vi "电源管理UI.vi"() -> ()   [LabVIEW 2016, in "环境动力单元.lvlib"]
uses:
  <vilib>/Utility/miscctls.llb/LVPointTypeDef.ctl
  <vilib>/Plasmionique/MB Master/MB_Master/MB_Master.lvclass
  <vilib>/Utility/config.llb/NI_LVConfig.lvlib
  <vilib>/ptbypt/NI_PtbyPt.lvlib
  API/AIRMAR WeatherCaster/AIRMAR WeatherCaster.lvlib
panel:
  out "门禁2状态":bool
  in  "停止":bool
  out "运行状态":string
  in  "采配水单次启动":bool
  out "充放电信息 2":T1 caption="充放电信息_KWH" {"总累计充电量" format="%.2f"; "当年累计充电量" format="%.2f"; "当月累计充电量" format="%.2f"; "当日累计充电量" format="%.2f"; "当年累计用电量" format="%.2f"; "当月累计用电量" format="%.2f"; "当日累计用电量" format="%.2f"}
  out "状态 2":string caption="状态"
  out "状态":string
  out "充放电信息":T1 caption="充放电信息_KWH" {"总累计充电量" format="%.2f"; "当年累计充电量" format="%.2f"; "当月累计充电量" format="%.2f"; "当日累计充电量" format="%.2f"; "当年累计用电量" format="%.2f"; "当月累计用电量" format="%.2f"; "当日累计用电量" format="%.2f"}
  out "通讯状态 3":bool
  out "通讯状态 2":bool
  out "通讯状态":bool
  in  "排气扇设置":bool
  in  "冰箱设置":bool
  in  "采配水设置":bool caption="报警设置"
  in  "MPPT-24 串口":refnum<visa-resource-name> caption="MPPT-24"
  in  "MPPT-24 启用":bool
  in  "MPPT-12 串口":refnum<visa-resource-name> caption="MPPT-12"
  in  "MPPT-12 启用":bool
  in  "报警设置":bool
  in  "排气扇":bool
  in  "冰箱":bool
  in  "排液阀":bool
  in  "采水泵":bool
  out "控制器信息 2":cluster{"设备温度℃":dbl} caption="控制器信息"
  out "直流负载信息 2":cluster{"负载电压V":dbl, "负载电流A":dbl, "负载功率W":dbl} caption="直流负载信息"
  out "蓄电池信息 2":T2 caption="蓄电池信息"
  out "阵列信息 2":cluster{"阵列电压V":dbl, "阵列电流A":dbl, "发电功率W":dbl} caption="阵列信息"
  out "控制器信息":cluster{"设备温度℃":dbl}
  out "直流负载信息":cluster{"负载电压V":dbl, "负载电流A":dbl, "负载功率W":dbl}
  out "蓄电池信息":T2
  out "阵列信息":cluster{"阵列电压V":dbl, "阵列电流A":dbl, "发电功率W":dbl}
  out "湿度":dbl format="%.0f %%RH"
  out "室温":dbl format="%.2f ℃"
  out "液位状态":bool
  out "门禁1状态":bool
  out "烟雾报警":bool
  out "水浸报警":bool
  in  "ZLAN启用":bool
  in  "模拟量配置":bool
  # "监控信息"
  # "MPPT-12"
  # "MPPT-24"
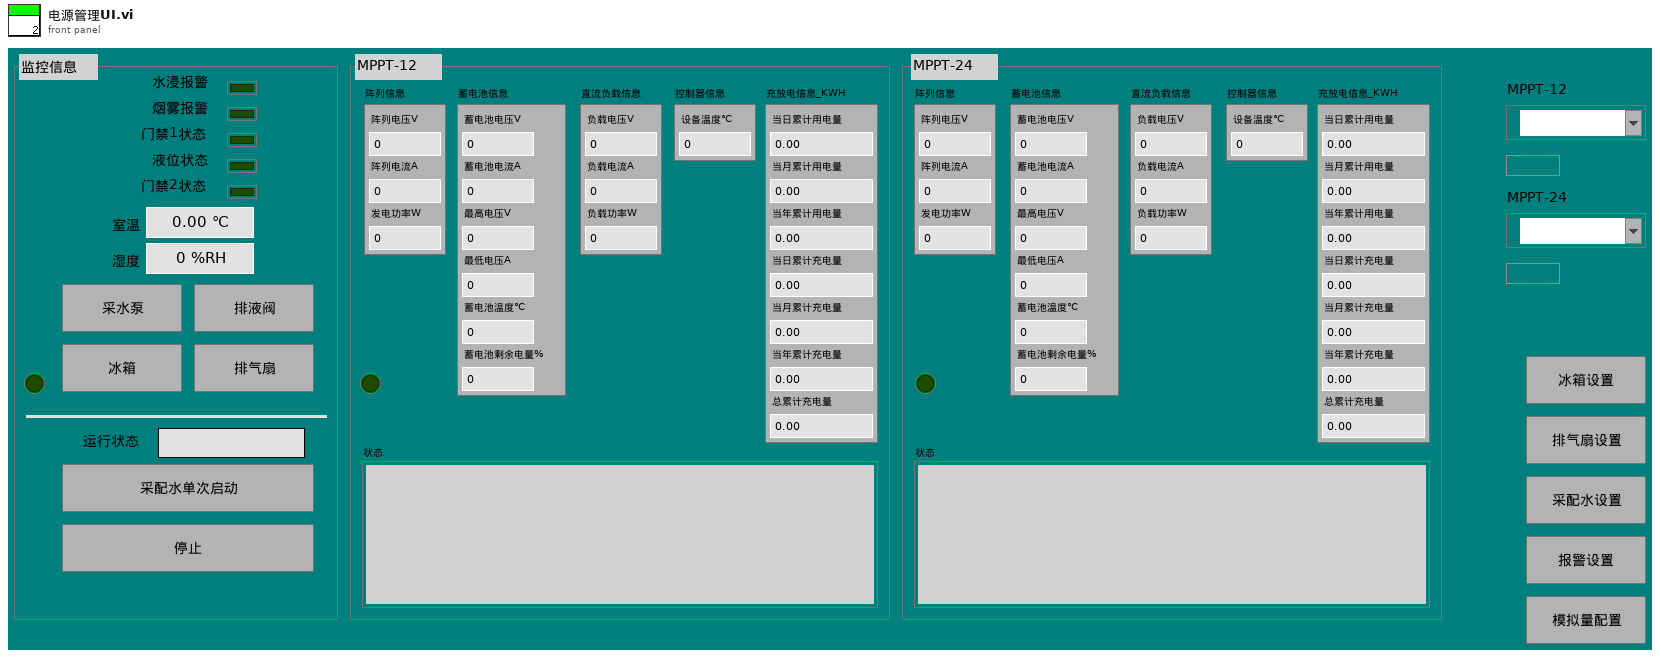
[diagram p1: front panel]
types:
  T1 = cluster{"当日累计用电量":sgl, "当月累计用电量":sgl, "当年累计用电量":sgl, "当日累计充电量":sgl, "当月累计充电量":sgl, "当年累计充电量":sgl, "总累计充电量":sgl}
  T2 = cluster{"蓄电池电压V":dbl, "蓄电池电流A":dbl, "最高电压V":dbl, "最低电压A":dbl, "蓄电池温度℃":dbl, "蓄电池剩余电量%":dbl}
  T3 = typedef "LVPointTypeDef.ctl" = cluster{"Horizontal":i16, "Vertical":i16}
  T4 = cluster{"蓄电池电压":dbl, "室温":dbl, "湿度":dbl, "水浸报警":bool, "烟雾报警":bool, "门禁1状态":bool, "门禁2状态":bool}
  T5 = cluster{"AD0":dbl, "AD1":dbl, "AD2":dbl, "AD3":dbl, "AD4":dbl, "AD5":dbl, "AD6":dbl, "AD7":dbl}
  T6 = typedef "NI_LVConfig.lvlib/Config Data RefNum.ctl" = refnum<k1>
  T7 = cluster{"时间":timestamp, "阵列电压_V":dbl, "阵列电流_A":dbl, "发电功率_W":dbl, "蓄电池电压_V":dbl, "蓄电池电流_A":dbl, "最高电压_V":dbl, "最低电压_A":dbl, "蓄电池温度_℃":dbl, "蓄电池剩余电量_%":dbl, "负载电压_V":dbl, "负载电流_A":dbl, "负载功率_W":dbl, "设备温度_℃":dbl, "当日累计用电量_KWH":dbl, "当月累计用电量_KWH":dbl, "当年累计用电量_KWH":dbl, "当日累计充电量_KWH":dbl, "当月累计充电量_KWH":dbl, "当年累计充电量_KWH":dbl, "总累计充电量_KWH":dbl}
  T8 = typedef "LVDateTimeRec.ctl" = cluster{"秒数的小数部分":dbl, "秒":i32, "分":i32, "时":i32, "日":i32, "月":i32, "年":i32, "天数（周）":i32, "天数（年）":i32, "DST":i32}
  T9 = cluster{"功能开关":enum16{"关闭", "开启"}, "开启时间":u16, "关闭时间":u16}
  T10 = cluster{"功能开关":enum16{"关闭", "开启"}, "排气扇开启温度":dbl, "排气扇关闭温度":dbl}
  T11 = cluster{"原始值最小值":dbl, "原始值最大值":dbl, "转换值最小值":dbl, "转换值最大值":dbl, "原始值最小值 2":dbl, "原始值最大值 2":dbl, "转换值最小值 2":dbl, "转换值最大值 2":dbl, "原始值最小值 3":dbl, "原始值最大值 3":dbl, "转换值最小值 3":dbl, "转换值最大值 3":dbl, "原始值最小值 4":dbl, "原始值最大值 4":dbl, "转换值最小值 4":dbl, "转换值最大值 4":dbl, "原始值最小值 5":dbl, "原始值最大值 5":dbl, "转换值最小值 5":dbl, "转换值最大值 5":dbl, "原始值最小值 6":dbl, "原始值最大值 6":dbl, "转换值最小值 6":dbl, "转换值最大值 6":dbl, "原始值最小值 7":dbl, "原始值最大值 7":dbl, "转换值最小值 7":dbl, "转换值最大值 7":dbl, "原始值最小值 8":dbl, "原始值最大值 8":dbl, "转换值最小值 8":dbl, "转换值最大值 8":dbl}
  T12 = enum8{"Enabled", "Disabled", "Disabled and Grayed Out"}
  T13 = cluster{"Registers[0]":u16, "Registers[1]":u16, "Registers[2]":u16, "Registers[3]":u16, "Registers[4]":u16, "Registers[5]":u16, "Registers[6]":u16, "Registers[7]":u16}
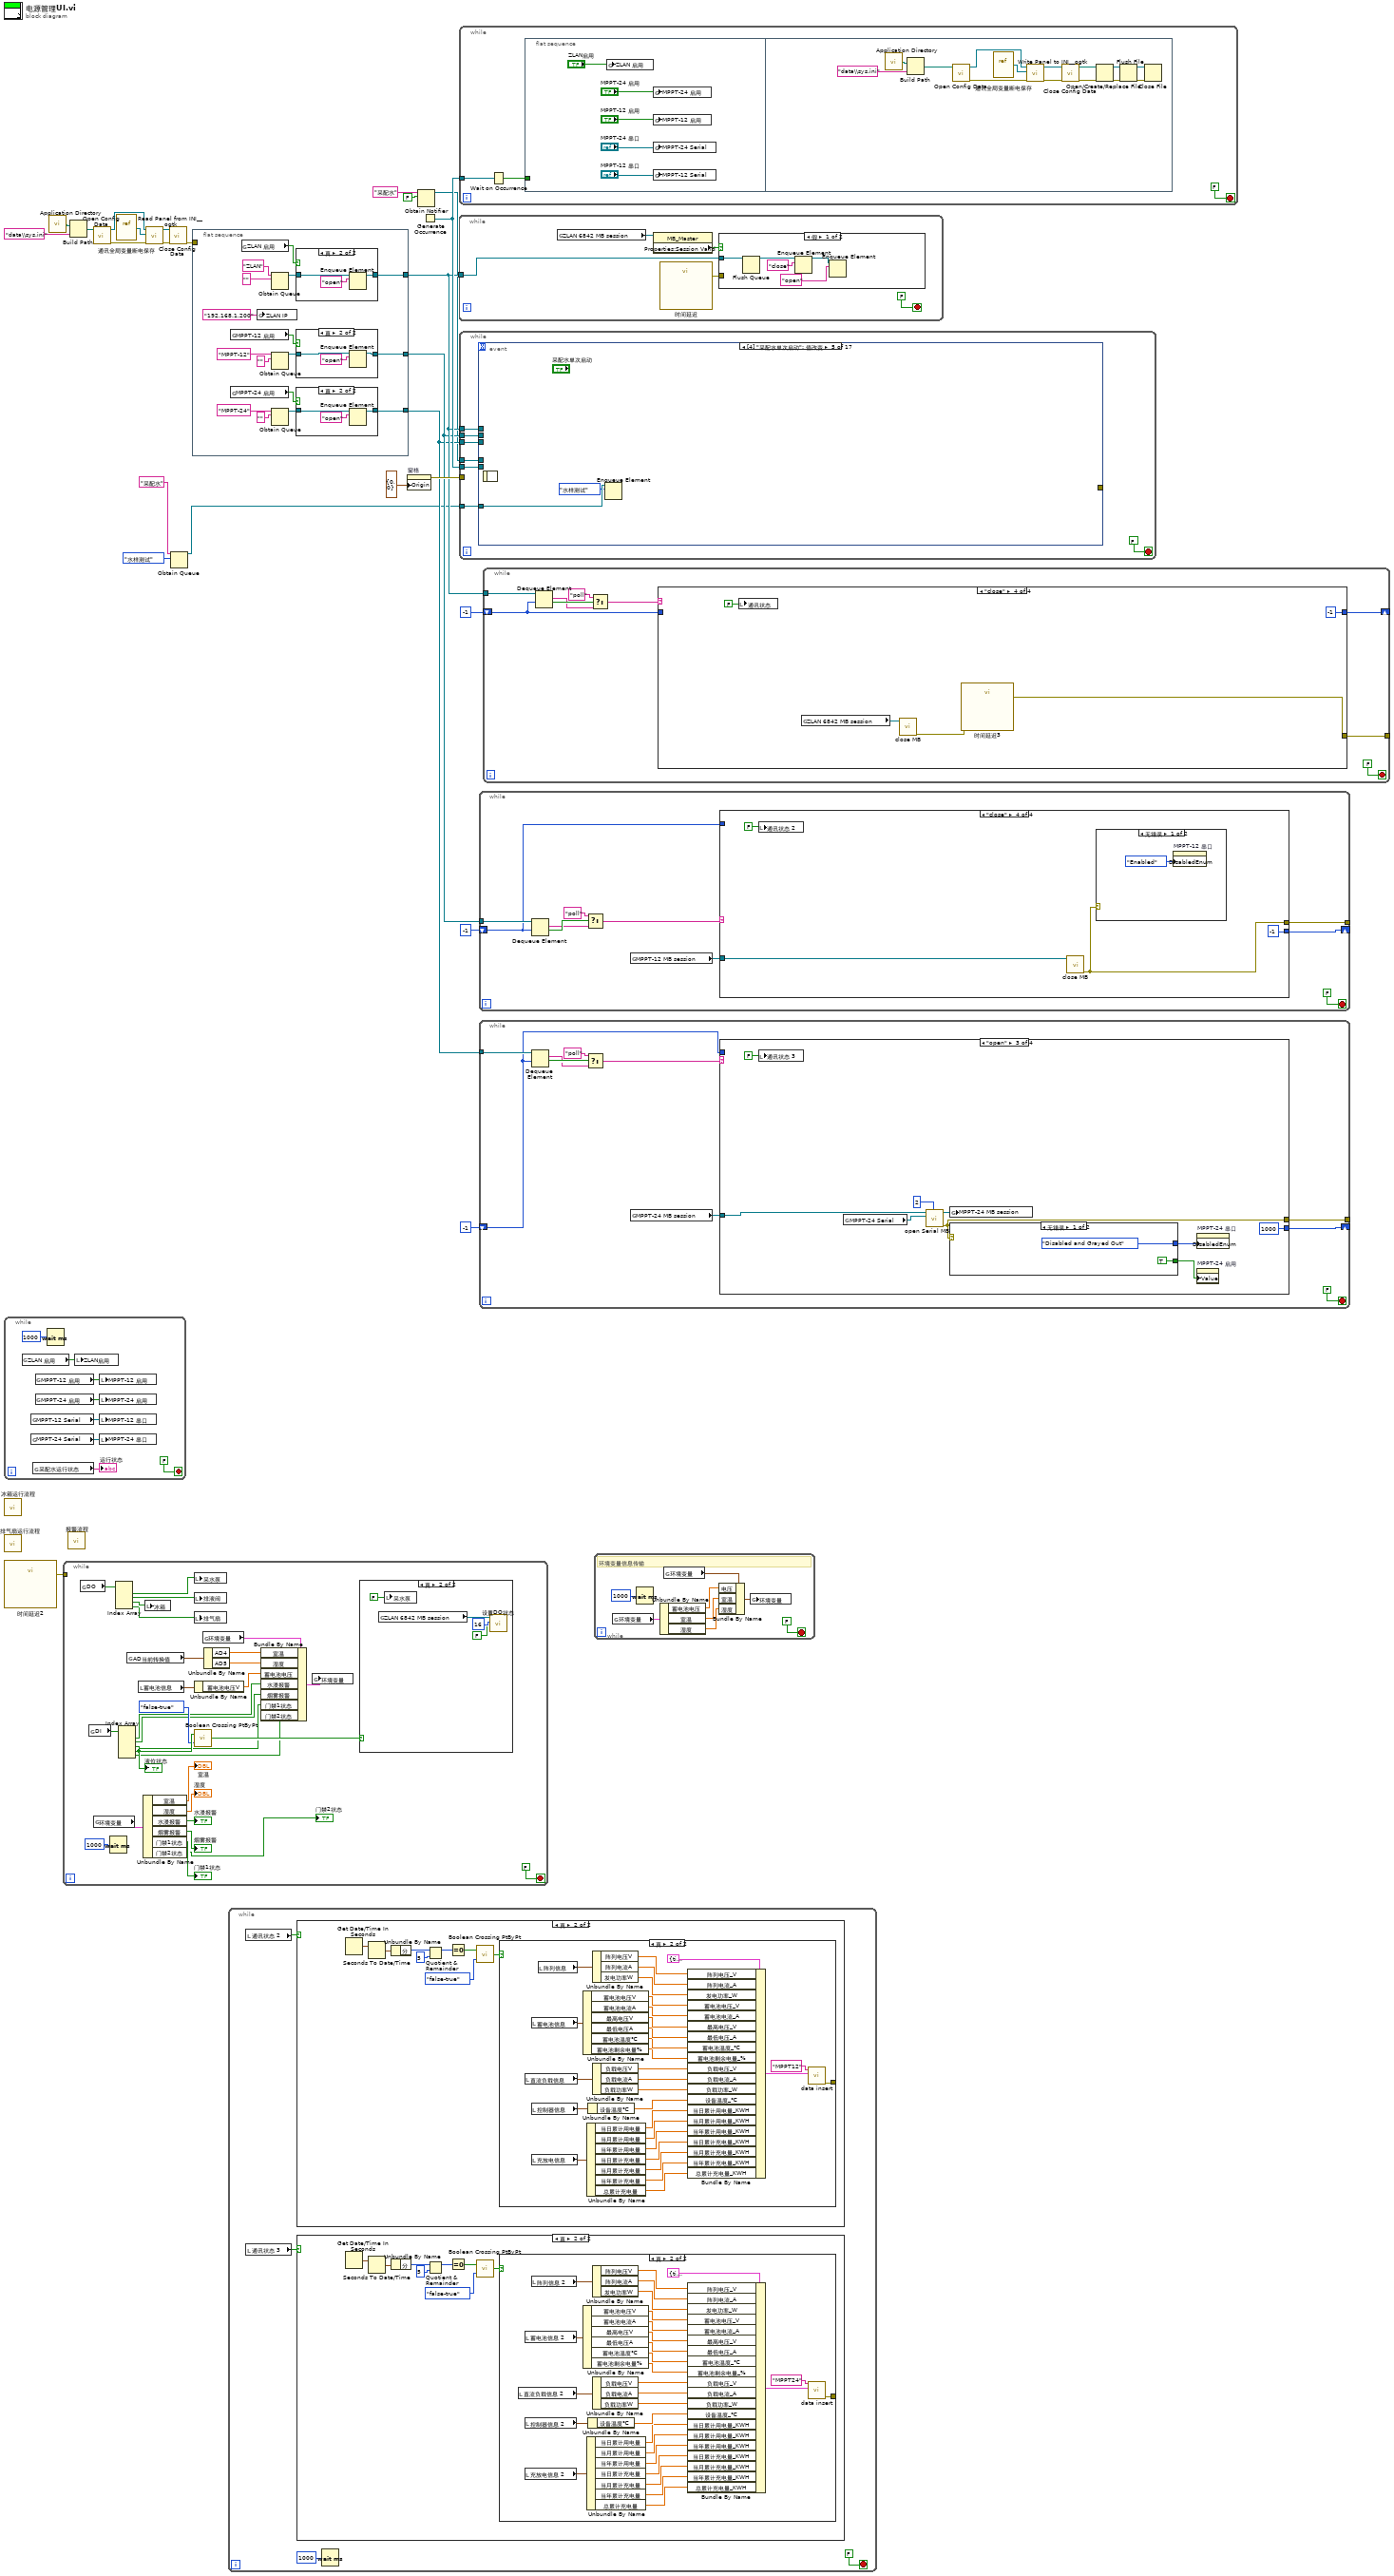
[diagram p0: block diagram]
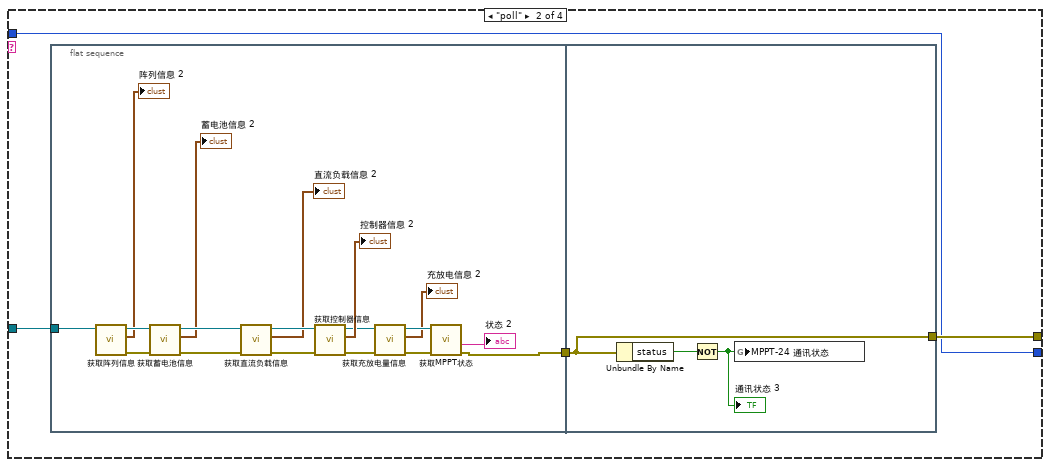
[diagram p7: hidden frame]
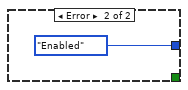
[diagram p8: hidden frame]
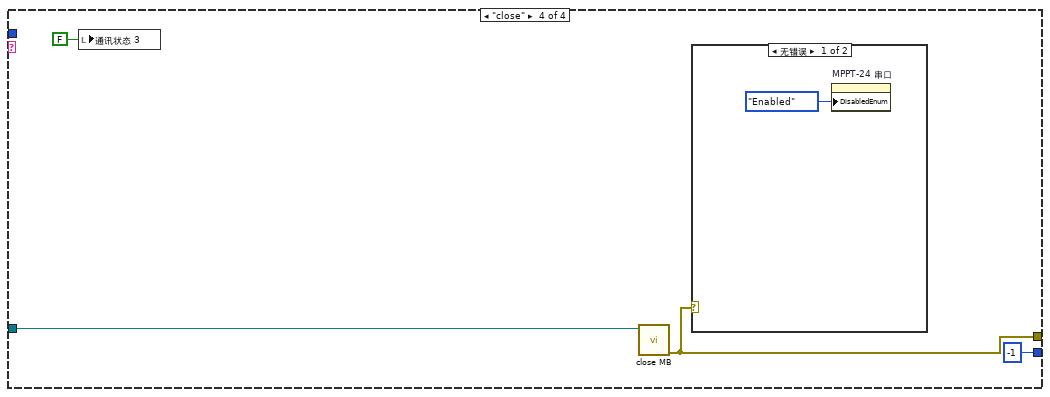
[diagram p9: hidden frame]
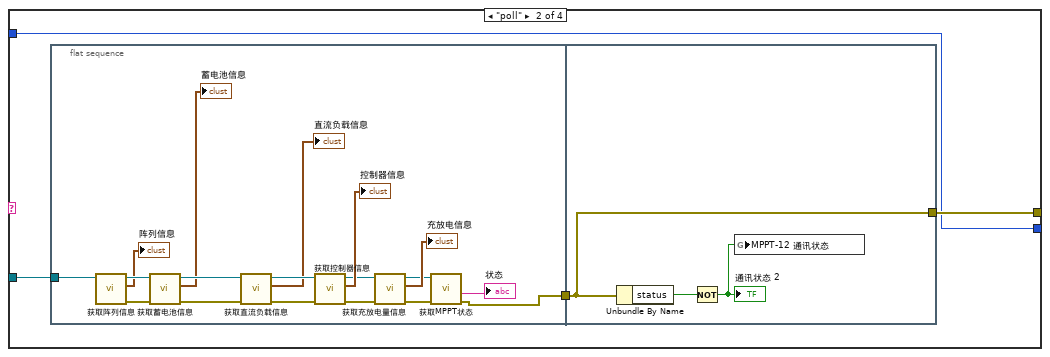
[diagram p12: hidden frame]
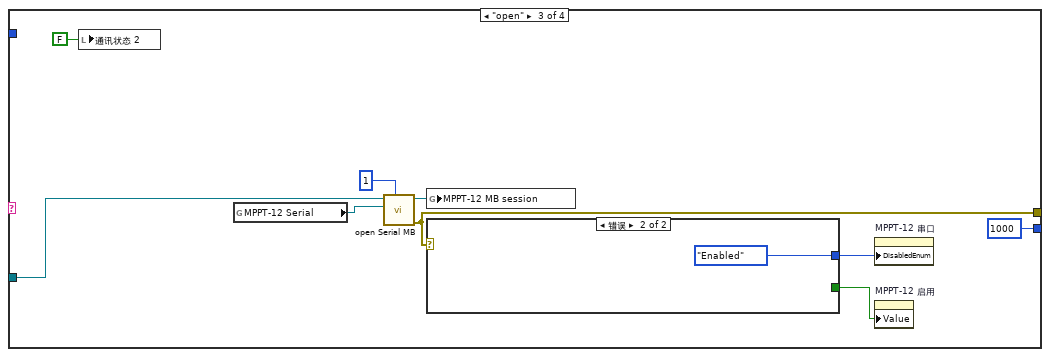
[diagram p13: hidden frame]
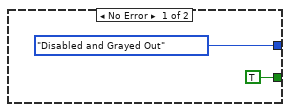
[diagram p14: hidden frame]
diagram:
  n1 = while {
    stop <- FALSE stop-if-true
    n2 = global read "通讯全局变量断电保存.vi" "ZLAN 启用"() -> (w31:bool)
    n3 = global read "通讯全局变量断电保存.vi" "MPPT-12 Serial"() -> (w28:refnum<visa-resource-name>)
    n4 = global read "通讯全局变量断电保存.vi" "MPPT-24 Serial"() -> (w27:refnum<visa-resource-name>)
    n5 = global read "通讯全局变量.vi" "采配水运行状态"() -> (→"运行状态":string)
    n6 = global read "通讯全局变量断电保存.vi" "MPPT-12 启用"() -> (w30:bool)
    n7 = global read "通讯全局变量断电保存.vi" "MPPT-24 启用"() -> (w29:bool)
    n8 = Wait (ms)(milliseconds to wait=u32 1000 ("等待时间（毫秒）")) -> ()  [unwired: 1 out]
    n9 = local write "ZLAN启用"(w31) -> ()
    n10 = local write "MPPT-12 启用"(w30) -> ()
    n11 = local write "MPPT-24 启用"(w29) -> ()
    n12 = local write "MPPT-12 串口"(w28) -> ()
    n13 = local write "MPPT-24 串口"(w27) -> ()
  }
  n14 = call "冰箱运行流程.vi"() -> ()  [unwired: 12 in]
  n15 = call "排气扇运行流程.vi"() -> ()  [unwired: 12 in]
  n16 = call "时间延迟2"() -> ("error out"=w15:errorcluster)  [unwired: 11 in]
  n17 = call <vilib>:"Application Directory.vi"() -> ("Application Directory"=w17:path)
  n18 = while {
    tunnel: w15 -> [_]
    stop <- FALSE stop-if-true
    n19 = global read "通讯全局变量.vi" "DO"() -> (w58:bool[])
    n20 = global read "通讯全局变量.vi" "DI"() -> (w59:bool[])
    n21 = global read "通讯全局变量.vi" "环境变量"() -> (w46:T4)
    n22 = Wait (ms)(milliseconds to wait=u32 1000 ("等待时间（毫秒）")) -> ()  [unwired: 1 out]
    n23 = Index Array(array=w58) -> (element #1=w57:bool, element #2=w56:bool, element #3=w55:bool, element #4=w54:bool)  [unwired: 4 in]
    n24 = Index Array(array=w59) -> (element #1=w41:bool, element #2=w40:bool, element #3=w39:bool, element #4=w53:bool, element #5=w35:bool)  [unwired: 5 in]
    "液位状态" <- w53
    n25 = global read "通讯全局变量.vi" "AD当前转换值"() -> (w61:T5)
    n26 = local read "蓄电池信息"() -> (w43:T2)
    n27 = Unbundle By Name(w46) -> ("室温"=→"室温":dbl, "湿度"=→"湿度":dbl, "水浸报警"=→"水浸报警":bool, "烟雾报警"=→"烟雾报警":bool, "门禁1状态"=→"门禁1状态":bool, "门禁2状态"=→"门禁2状态":bool)
    n28 = local write "冰箱"(w55) -> ()
    n29 = local write "采水泵"(w57) -> ()
    n30 = local write "排液阀"(w56) -> ()
    n31 = local write "排气扇"(w54) -> ()
    n32 = Unbundle By Name(w43) -> ("蓄电池电压V"=w42:dbl)
    n33 = call <vilib>:"Boolean Crossing PtByPt.vi"("direction"=enum16{"either", "false-true", "true-false"}."false-true", "input"=w53) -> ("crossing"=w52:bool)  [unwired: 1 in]
    n34 = global read "通讯全局变量.vi" "环境变量"() -> (w50:T4)
    n35 = Unbundle By Name(w61) -> ("AD4"=w49:dbl, "AD5"=w48:dbl)
    n36 = Bundle By Name(cluster=w50, "室温"=w49, "湿度"=w48, "蓄电池电压"=w42, "水浸报警"=w41, "烟雾报警"=w40, "门禁1状态"=w39, "门禁2状态"=w35) -> (w47:T4)
    n37 = global write "通讯全局变量.vi" "环境变量"(w47) -> ()
    n38 = case shown="真" w52 {
      frame False {
      }
      frame True {
        n39 = global read "通讯全局变量.vi" "ZLAN 6842 MB session"() -> (w66:refnum<class "MB_Master.lvclass">)
        n40 = local write "采水泵"(FALSE ("采水泵")) -> ()
        n41 = call "设置DO状态.vi"("value"=FALSE, "address"=u16 16, "MB session in"=w66) -> ()  [unwired: 7 in, 2 out]
      }
    }
  }
  n42 = call "报警流程.vi"() -> ()  [unwired: 12 in]
  n43 = Build Path(base path=w17, name or relative path="data\\sys.ini" ("名称或相对路径")) -> (appended path=w19:path)
  n44 = call <vilib>:"Open Config Data.vi"("configuration file path"=w19) -> ("error out"=w23:errorcluster, "refnum"=w20:T6)  [unwired: 8 in, 1 out]
  n45 = vi-ref "通讯全局变量断电保存.vi"() -> (w21:refnum<vi>)
  n46 = call <userlib>:"Read Panel from INI__ogtk.vi"("error in (no error)"=w23, "VI ref"=w21, "refnum"=w20) -> ("error out"=w16:errorcluster, "refnum out"=w22:T6)  [unwired: 7 in]
  n47 = call <vilib>:"Close Config Data.vi"("error in (no error)"=w16, "refnum"=w22) -> ("error out"=w12:errorcluster)  [unwired: 8 in, 1 out]
  n48 = Obtain Queue(name (unnamed)="采配水" ("名称（未命名）"), element data type=enum16{"水样测试", "加标回收"}."水样测试" ("启动类型")) -> (queue out=w1:refnum<queue>)  [unwired: 3 in, 2 out]
  n49 = flat-sequence {
    tunnel: [w79] -> w11
    tunnel: w12 -> [_]
    tunnel: [w73] -> w9
    tunnel: [w68] -> w7
    frame #0 {
      n50 = global read "通讯全局变量断电保存.vi" "MPPT-12 启用"() -> (w77:bool)
      n51 = global read "通讯全局变量断电保存.vi" "MPPT-24 启用"() -> (w69:bool)
      n52 = global read "通讯全局变量断电保存.vi" "ZLAN 启用"() -> (w78:bool)
      n53 = global write "通讯全局变量断电保存.vi" "ZLAN IP"("192.168.1.200" ("ZLAN IP")) -> ()
      n54 = Obtain Queue(name (unnamed)="ZLAN" ("名称（未命名）"), element data type="") -> (queue out=w80:refnum<queue>)  [unwired: 3 in, 2 out]
      n55 = Obtain Queue(name (unnamed)="MPPT-12" ("名称（未命名）"), element data type="") -> (queue out=w76:refnum<queue>)  [unwired: 3 in, 2 out]
      n56 = Obtain Queue(name (unnamed)="MPPT-24" ("名称（未命名）"), element data type="") -> (queue out=w70:refnum<queue>)  [unwired: 3 in, 2 out]
      n57 = case shown="真" w78 {
        tunnel: w80 -> [w91 w94]
        tunnel: [w91 w92] -> w79
        frame False {
        }
        frame True {
          n58 = Enqueue Element(queue=w94, element="open" ("元素")) -> (queue out=w92:refnum<queue>)  [unwired: 2 in, 2 out]
        }
      }
      n59 = case shown="真" w77 {
        tunnel: w76 -> [w87 w90]
        tunnel: [w87 w88] -> w73
        frame False {
        }
        frame True {
          n60 = Enqueue Element(queue=w90, element="open" ("元素")) -> (queue out=w88:refnum<queue>)  [unwired: 2 in, 2 out]
        }
      }
      n61 = case shown="真" w69 {
        tunnel: w70 -> [w83 w86]
        tunnel: [w83 w84] -> w68
        frame False {
        }
        frame True {
          n62 = Enqueue Element(queue=w86, element="open" ("元素")) -> (queue out=w84:refnum<queue>)  [unwired: 2 in, 2 out]
        }
      }
    }
  }
  n63 = while {
    stop <- FALSE stop-if-true
    n64 = local read "通讯状态 2"() -> (w97:bool)
    n65 = local read "通讯状态 3"() -> (w96:bool)
    n66 = case shown="真" w97 {
      frame False {
      }
      frame True {
        n67 = Get Date/Time In Seconds() -> (seconds since 1Jan1904=w143:timestamp)
        n68 = Seconds To Date/Time(time stamp (now)=w143) -> (date time rec=w142:T8)  [unwired: 1 in]
        n69 = Unbundle By Name(w142) -> ("分"=w141:i32)
        n70 = Quotient & Remainder(x=w141, y=5) -> (x-y*floor(x/y)=w139:i32)  [unwired: 1 out]
        n71 = Equal To 0?(x=w139) -> (x = 0?=w138:bool)
        n72 = call <vilib>:"Boolean Crossing PtByPt.vi"("direction"=enum16{"either", "false-true", "true-false"}."false-true", "input"=w138) -> ("crossing"=w136:bool)  [unwired: 1 in]
        n73 = case shown="真" w136 {
          tunnel: [_ w144] -> _
          frame False {
          }
          frame True {
            n74 = local read "直流负载信息"() -> (w158:cluster{"负载电压V":dbl, "负载电流A":dbl, "负载功率W":dbl})
            n75 = local read "蓄电池信息"() -> (w165:T2)
            n76 = local read "控制器信息"() -> (w154:cluster{"设备温度℃":dbl})
            n77 = local read "充放电信息"() -> (w152:T1)
            n78 = local read "阵列信息"() -> (w169:cluster{"阵列电压V":dbl, "阵列电流A":dbl, "发电功率W":dbl})
            n79 = Unbundle By Name(w165) -> ("蓄电池电压V"=w164:dbl, "蓄电池电流A"=w163:dbl, "最高电压V"=w162:dbl, "最低电压A"=w161:dbl, "蓄电池温度℃"=w160:dbl, "蓄电池剩余电量%"=w159:dbl)
            n80 = Unbundle By Name(w152) -> ("当日累计用电量"=w151:sgl, "当月累计用电量"=w150:sgl, "当年累计用电量"=w149:sgl, "当日累计充电量"=w148:sgl, "当月累计充电量"=w147:sgl, "当年累计充电量"=w146:sgl, "总累计充电量"=w145:sgl)
            n81 = Unbundle By Name(w154) -> ("设备温度℃"=w153:dbl)
            n82 = Unbundle By Name(w169) -> ("阵列电压V"=w168:dbl, "阵列电流A"=w167:dbl, "发电功率W"=w166:dbl)
            n83 = Unbundle By Name(w158) -> ("负载电压V"=w157:dbl, "负载电流A"=w156:dbl, "负载功率W"=w155:dbl)
            n84 = Bundle By Name(cluster=T7 {"时间"=timestamp(0 s since 1904-01-01), "阵列电压_V"=0.0, "阵列电流_A"=0.0, "发电功率_W"=0.0, "蓄电池电压_V"=0.0, "蓄电池电流_A"=0.0, "最高电压_V"=0.0, "最低电压_A"=0.0, "蓄电池温度_℃"=0.0, "蓄电池剩余电量_%"=0.0, "负载电压_V"=0.0, "负载电流_A"=0.0, "负载功率_W"=0.0, "设备温度_℃"=0.0, "当日累计用电量_KWH"=0.0, "当月累计用电量_KWH"=0.0, "当年累计用电量_KWH"=0.0, "当日累计充电量_KWH"=0.0, "当月累计充电量_KWH"=0.0, "当年累计充电量_KWH"=0.0, "总累计充电量_KWH"=0.0} ("data in"), "阵列电压_V"=w168, "阵列电流_A"=w167, "发电功率_W"=w166, "蓄电池电压_V"=w164, "蓄电池电流_A"=w163, "最高电压_V"=w162, "最低电压_A"=w161, "蓄电池温度_℃"=w160, "蓄电池剩余电量_%"=w159, "负载电压_V"=w157, "负载电流_A"=w156, "负载功率_W"=w155, "设备温度_℃"=w153, "当日累计用电量_KWH"=w151, "当月累计用电量_KWH"=w150, "当年累计用电量_KWH"=w149, "当日累计充电量_KWH"=w148, "当月累计充电量_KWH"=w147, "当年累计充电量_KWH"=w146, "总累计充电量_KWH"=w145) -> (w170:T7)
            n85 = call "data insert.vi"("data in"=w170, "table"="MPPT12") -> ("error out"=w144:errorcluster)  [unwired: 9 in]
          }
        }
      }
    }
    n86 = case shown="真" w96 {
      frame False {
      }
      frame True {
        n87 = Get Date/Time In Seconds() -> (seconds since 1Jan1904=w99:timestamp)
        n88 = Seconds To Date/Time(time stamp (now)=w99) -> (date time rec=w100:T8)  [unwired: 1 in]
        n89 = Unbundle By Name(w100) -> ("分"=w101:i32)
        n90 = Quotient & Remainder(x=w101, y=5) -> (x-y*floor(x/y)=w103:i32)  [unwired: 1 out]
        n91 = Equal To 0?(x=w103) -> (x = 0?=w104:bool)
        n92 = call <vilib>:"Boolean Crossing PtByPt.vi"("direction"=enum16{"either", "false-true", "true-false"}."false-true", "input"=w104) -> ("crossing"=w106:bool)  [unwired: 1 in]
        n93 = case shown="真" w106 {
          tunnel: [_ w107] -> _
          frame False {
          }
          frame True {
            n94 = local read "直流负载信息 2"() -> (w121:cluster{"负载电压V":dbl, "负载电流A":dbl, "负载功率W":dbl})
            n95 = local read "蓄电池信息 2"() -> (w128:T2)
            n96 = local read "控制器信息 2"() -> (w117:cluster{"设备温度℃":dbl})
            n97 = local read "充放电信息 2"() -> (w115:T1)
            n98 = local read "阵列信息 2"() -> (w132:cluster{"阵列电压V":dbl, "阵列电流A":dbl, "发电功率W":dbl})
            n99 = Unbundle By Name(w128) -> ("蓄电池电压V"=w127:dbl, "蓄电池电流A"=w126:dbl, "最高电压V"=w125:dbl, "最低电压A"=w124:dbl, "蓄电池温度℃"=w123:dbl, "蓄电池剩余电量%"=w122:dbl)
            n100 = Unbundle By Name(w115) -> ("当日累计用电量"=w114:sgl, "当月累计用电量"=w113:sgl, "当年累计用电量"=w112:sgl, "当日累计充电量"=w111:sgl, "当月累计充电量"=w110:sgl, "当年累计充电量"=w109:sgl, "总累计充电量"=w108:sgl)
            n101 = Unbundle By Name(w117) -> ("设备温度℃"=w116:dbl)
            n102 = Unbundle By Name(w132) -> ("阵列电压V"=w131:dbl, "阵列电流A"=w130:dbl, "发电功率W"=w129:dbl)
            n103 = Unbundle By Name(w121) -> ("负载电压V"=w120:dbl, "负载电流A"=w119:dbl, "负载功率W"=w118:dbl)
            n104 = Bundle By Name(cluster=T7 {"时间"=timestamp(0 s since 1904-01-01), "阵列电压_V"=0.0, "阵列电流_A"=0.0, "发电功率_W"=0.0, "蓄电池电压_V"=0.0, "蓄电池电流_A"=0.0, "最高电压_V"=0.0, "最低电压_A"=0.0, "蓄电池温度_℃"=0.0, "蓄电池剩余电量_%"=0.0, "负载电压_V"=0.0, "负载电流_A"=0.0, "负载功率_W"=0.0, "设备温度_℃"=0.0, "当日累计用电量_KWH"=0.0, "当月累计用电量_KWH"=0.0, "当年累计用电量_KWH"=0.0, "当日累计充电量_KWH"=0.0, "当月累计充电量_KWH"=0.0, "当年累计充电量_KWH"=0.0, "总累计充电量_KWH"=0.0} ("data in"), "阵列电压_V"=w131, "阵列电流_A"=w130, "发电功率_W"=w129, "蓄电池电压_V"=w127, "蓄电池电流_A"=w126, "最高电压_V"=w125, "最低电压_A"=w124, "蓄电池温度_℃"=w123, "蓄电池剩余电量_%"=w122, "负载电压_V"=w120, "负载电流_A"=w119, "负载功率_W"=w118, "设备温度_℃"=w116, "当日累计用电量_KWH"=w114, "当月累计用电量_KWH"=w113, "当年累计用电量_KWH"=w112, "当日累计充电量_KWH"=w111, "当月累计充电量_KWH"=w110, "当年累计充电量_KWH"=w109, "总累计充电量_KWH"=w108) -> (w133:T7)
            n105 = call "data insert.vi"("data in"=w133, "table"="MPPT24") -> ("error out"=w107:errorcluster)  [unwired: 9 in]
          }
        }
      }
    }
    n106 = Wait (ms)(milliseconds to wait=u32 1000 ("等待时间（毫秒）")) -> ()  [unwired: 1 out]
  }
  n107 = property on="窗格" class="Pane"("Origin"=T3 {"Horizontal"=0, "Vertical"=0} ("原点")) -> (error out=w24:errorcluster)  [unwired: 2 in, 1 out]
  n108 = Obtain Notifier(name (unnamed)="采配水" ("名称（未命名）"), notification data type=FALSE) -> (notifier out=w4:refnum<notifier>)  [unwired: 2 in, 2 out]
  n109 = Generate Occurrence() -> (w13:refnum<k4>)
  n110 = while {
    tunnel: w11 -> [w175]
    stop <- FALSE stop-if-true
    n111 = global read "通讯全局变量.vi" "ZLAN 6842 MB session"() -> (w177:refnum<class "MB_Master.lvclass">)
    n112 = property class="MB_Master"(reference=w177) -> ("Properties:Session Valid"=w176:bool)  [unwired: 1 in, 2 out]
    n113 = call "时间延迟"() -> ("error out"=w174:errorcluster)  [unwired: 11 in]
    n114 = case shown="假" w176 {
      tunnel: w175 -> [w182 _]
      tunnel: w174 -> [_ _]
      frame False {
        n115 = Flush Queue(queue=w182) -> (queue out=w180:refnum<queue>)  [unwired: 1 in, 2 out]
        n116 = Enqueue Element(queue=w180, element="close") -> (queue out=w179:refnum<queue>)  [unwired: 2 in, 2 out]
        n117 = Enqueue Element(queue=w179, element="open") -> ()  [unwired: 2 in, 3 out]
      }
      frame True {
      }
    }
  }
  n118 = while {
    tunnel: w13 -> [w184]
    stop <- FALSE stop-if-true
    n119 = Wait on Occurrence(2:w184) -> (0:w183:bool)  [unwired: 2 in]
    n120 = flat-sequence {
      tunnel: w183 -> [_]
      frame #0 {
        n121 = global write "通讯全局变量断电保存.vi" "ZLAN 启用"("ZLAN启用") -> ()
        n122 = global write "通讯全局变量断电保存.vi" "MPPT-24 启用"("MPPT-24 启用") -> ()
        n123 = global write "通讯全局变量断电保存.vi" "MPPT-12 启用"("MPPT-12 启用") -> ()
        n124 = global write "通讯全局变量断电保存.vi" "MPPT-24 Serial"("MPPT-24 串口") -> ()
        n125 = global write "通讯全局变量断电保存.vi" "MPPT-12 Serial"("MPPT-12 串口") -> ()
      }
      frame #1 {
        n126 = call <vilib>:"Application Directory.vi"() -> ("Application Directory"=w204:path)
        n127 = Build Path(base path=w204, name or relative path="data\\sys.ini" ("名称或相对路径")) -> (appended path=w202:path)
        n128 = call <vilib>:"Open Config Data.vi"("configuration file path"=w202) -> ("error out"=w198:errorcluster, "refnum"=w201:T6)  [unwired: 8 in, 1 out]
        n129 = vi-ref "通讯全局变量断电保存.vi"() -> (w200:refnum<vi>)
        n130 = call <userlib>:"Write Panel to INI__ogtk.vi"("error in (no error)"=w198, "VI ref"=w200, "refnum"=w201) -> ("error out"=w197:errorcluster, "refnum out"=w199:T6)  [unwired: 7 in]
        n131 = call <vilib>:"Close Config Data.vi"("error in (no error)"=w197, "refnum"=w199) -> ("error out"=w192:errorcluster, "file path"=w191:path)  [unwired: 8 in]
        n132 = Open/Create/Replace File(file path (use dialog)=w191, error in=w192) -> (refnum out=w195:refnum<file>, error out=w196:errorcluster)  [unwired: 4 in, 1 out]
        n133 = Flush File(refnum=w195, error in=w196) -> (refnum out=w194:refnum<file>, error out=w193:errorcluster)
        n134 = Close File(refnum=w194, error in=w193) -> ()  [unwired: 2 out]
      }
    }
  }
  n135 = while {
    tunnel: w24 -> [_]
    tunnel: w11 -> [w210]
    tunnel: w13 -> [w209]
    tunnel: w9 -> [w208]
    tunnel: w7 -> [w207]
    tunnel: w4 -> [w206]
    tunnel: w1 -> [w205]
    stop <- FALSE stop-if-true
    n136 = event shown="[4] \"采配水单次启动\": 值改变" {
      selector: _ -> [_ _ _ _ _ _ _ _ _ _ _ _ _ _ _ _ _]
      dyn-events: _ -> [_ _ _ _ _ _ _ _ _ _ _ _ _ _ _ _ _]
      timeout: _ -> [_ _ _ _ _ _ _ _ _ _ _ _ _ _ _ _ _]
      tunnel: w210 -> [_ _ _ _ _ _ _ _ _ _ _ w252 _ _ _ _ _]
      tunnel: w209 -> [_ _ _ _ _ _ _ _ _ _ _ w254 w260 w266 w267 w268 _]
      tunnel: [_ _ _ _ _ _ _ w221 w227 w233 w242 _ _ _ _ _ _] -> _
      tunnel: w208 -> [_ _ _ _ _ _ _ _ _ _ _ _ w255 _ _ _ _]
      tunnel: w207 -> [_ _ _ _ _ _ _ _ _ _ _ _ _ w261 _ _ _]
      tunnel: w206 -> [_ _ _ _ _ w218 _ _ _ _ _ _ _ _ _ _ _]
      tunnel: w205 -> [_ _ _ _ w213 _ _ _ _ _ _ _ _ _ _ _ _]
      event Timeout {
        n137 = event-data() -> ()  [unwired: 1 in, 3 out]
      }
      event "冰箱设置": Value Change {
        n138 = event-data() -> ()  [unwired: 1 in, 6 out]
        n139 = call "冰箱设置.vi"() -> ()  [unwired: 12 in]
      }
      event "排气扇设置": Value Change {
        n140 = event-data() -> ()  [unwired: 1 in, 6 out]
        n141 = call "风扇设置.vi"() -> ()  [unwired: 12 in]
      }
      event "报警设置": Value Change {
        n142 = event-data() -> ()  [unwired: 1 in, 6 out]
        n143 = call "报警设置.vi"() -> ()  [unwired: 12 in]
      }
      event "采配水单次启动": Value Change {
        n144 = event-data() -> ()  [unwired: 1 in, 1 out]
        n145 = Enqueue Element(queue=w213, element=enum16{"水样测试", "加标回收"}."水样测试" ("元素")) -> ()  [unwired: 2 in, 3 out]
      }
      event "停止": Value Change {
        n146 = event-data() -> ()  [unwired: 1 in, 6 out]
        n147 = Send Notification(notification=TRUE ("通知"), notifier=w218) -> ()  [unwired: 1 in, 2 out]
        n148 = property on="采水泵" class="Bool (严格)"("Val(Sgnl)"=FALSE ("值(信号)")) -> (error out=w215:errorcluster)  [unwired: 2 in, 1 out]
        n149 = property on="排液阀" class="Bool (严格)"(error in=w215, "Val(Sgnl)"=FALSE ("值(信号)")) -> ()  [unwired: 1 in, 2 out]
      }
      event "采配水设置": Value Change {
        n150 = event-data() -> ()  [unwired: 1 in, 6 out]
        n151 = call "采配水参数设置.vi"() -> ()  [unwired: 12 in]
      }
      event "采水泵": Value Change {
        n152 = event-data() -> ("NewVal"=w222:bool)  [unwired: 1 in, 5 out]
        n153 = local read "液位状态"() -> (w219:bool)
        n154 = Not(x=w219) -> (.not. x?=w220:bool)
        n155 = case shown="假" w220 {
          tunnel: w222 -> [_ w224]
          tunnel: [_ w223] -> w221
          frame False {
          }
          frame True {
            n156 = global read "通讯全局变量.vi" "ZLAN 6842 MB session"() -> (w226:refnum<class "MB_Master.lvclass">)
            n157 = call "设置DO状态.vi"("value"=w224, "address"=u16 16, "MB session in"=w226) -> ("error out"=w223:errorcluster)  [unwired: 7 in, 1 out]
          }
        }
      }
      event "排液阀": Value Change {
        n158 = event-data() -> ("NewVal"=w228:bool)  [unwired: 1 in, 5 out]
        n159 = global read "通讯全局变量.vi" "ZLAN 6842 MB session"() -> (w230:refnum<class "MB_Master.lvclass">)
        n160 = call "设置DO状态.vi"("value"=w228, "address"=u16 17, "MB session in"=w230) -> ("error out"=w227:errorcluster)  [unwired: 7 in, 1 out]
      }
      event "冰箱": Value Change {
        n161 = event-data() -> ("NewVal"=w234:bool)  [unwired: 1 in, 5 out]
        n162 = global read "通讯全局变量断电保存.vi" "冰箱参数"() -> (w232:T9)
        n163 = Unbundle By Name(w232) -> ("功能开关"=w231:enum16{"关闭", "开启"})
        n164 = case shown="\"关闭\", 默认" w231 {
          tunnel: w234 -> [w236 _]
          tunnel: [w235 _] -> w233
          frame "关闭", Default {
            n165 = global read "通讯全局变量.vi" "ZLAN 6842 MB session"() -> (w238:refnum<class "MB_Master.lvclass">)
            n166 = call "设置DO状态.vi"("value"=w236, "address"=u16 18, "MB session in"=w238) -> ("error out"=w235:errorcluster)  [unwired: 7 in, 1 out]
          }
          frame "开启" {
            n167 = One Button Dialog(message="无法设置，只有 冰箱设置-功能开关 处于关闭状态才可以设置！" ("消息")) -> ()  [unwired: 1 in, 1 out]
          }
        }
      }
      event "排气扇": Value Change {
        n168 = event-data() -> ("NewVal"=w243:bool)  [unwired: 1 in, 5 out]
        n169 = global read "通讯全局变量断电保存.vi" "排气扇参数"() -> (w241:T10)
        n170 = Unbundle By Name(w241) -> ("功能开关"=w240:enum16{"关闭", "开启"})
        n171 = case shown="\"关闭\", 默认" w240 {
          tunnel: w243 -> [w245 _]
          tunnel: [w244 _] -> w242
          frame "关闭", Default {
            n172 = global read "通讯全局变量.vi" "ZLAN 6842 MB session"() -> (w247:refnum<class "MB_Master.lvclass">)
            n173 = call "设置DO状态.vi"("value"=w245, "address"=u16 19, "MB session in"=w247) -> ("error out"=w244:errorcluster)  [unwired: 7 in, 1 out]
          }
          frame "开启" {
            n174 = One Button Dialog(message="无法设置，只有 排气扇设置-功能开关 处于关闭状态才可以设置！" ("消息")) -> ()  [unwired: 1 in, 1 out]
          }
        }
      }
      event "ZLAN启用": Value Change {
        n175 = event-data() -> ("NewVal"=w253:bool)  [unwired: 1 in]
        n176 = Set Occurrence(w254) -> ()
        n177 = Select(t="open", s=w253, f="close") -> (s? t:f=w250:string)
        n178 = Enqueue Element(queue=w252, element=w250) -> ()  [unwired: 2 in, 3 out]
      }
      event "MPPT-12 启用": Value Change {
        n179 = event-data() -> ("NewVal"=w259:bool)  [unwired: 1 in]
        n180 = Set Occurrence(w260) -> ()
        n181 = Select(t="open", s=w259, f="close") -> (s? t:f=w257:string)
        n182 = Enqueue Element(queue=w255, element=w257) -> ()  [unwired: 2 in, 3 out]
      }
      event "MPPT-24 启用": Value Change {
        n183 = event-data() -> ("NewVal"=w265:bool)  [unwired: 1 in]
        n184 = Set Occurrence(w266) -> ()
        n185 = Select(t="open", s=w265, f="close") -> (s? t:f=w263:string)
        n186 = Enqueue Element(queue=w261, element=w263) -> ()  [unwired: 2 in, 3 out]
      }
      event "MPPT-12 串口": Value Change {
        n187 = event-data() -> ()  [unwired: 1 in, 5 out]
        n188 = Set Occurrence(w267) -> ()
      }
      event "MPPT-24 串口": Value Change {
        n189 = event-data() -> ()  [unwired: 1 in, 5 out]
        n190 = Set Occurrence(w268) -> ()
      }
      event "模拟量配置": Value Change {
        n191 = event-data() -> ()  [unwired: 1 in, 6 out]
        n192 = global read "通讯全局变量断电保存.vi" "工程量转换"() -> (w269:T11)
        n193 = call "模拟量配置.vi"("工程量转换"=w269) -> ()  [unwired: 11 in]
      }
    }
  }
  n194 = while {
    tunnel: w9 -> [w279]
    tunnel: [w271] -> _
    shift-right: [w272] -> _
    shift-left: -1 ("超时毫秒(-1)") -> [w273]
    stop <- FALSE stop-if-true
    n195 = Dequeue Element(queue=w279, timeout in ms (-1)=w273) -> (element=w276:string, timed out?=w278:bool)  [unwired: 1 in, 2 out]
    n196 = Select(t="poll" ("元素"), s=w278, f=w276) -> (s? t:f=w275:string)
    n197 = global read "通讯全局变量.vi" "MPPT-12 MB session"() -> (w270:refnum<class "MB_Master.lvclass">)
    n198 = case shown="\"close\"" w275 {
      tunnel: [_ w284 w308 w318] -> w271
      tunnel: w273 -> [w280 w282 _ _]
      tunnel: [w280 w282 1000 ("超时毫秒(-1)") -1 ("超时毫秒(-1)")] -> w272
      tunnel: w270 -> [_ w281 w309 w319]
      frame Default {
      }
      frame "poll" {
        n199 = flat-sequence {
          tunnel: [w286] -> w283
          tunnel: w281 -> [w296]
          tunnel: [w304] -> w284
          tunnel: w283 -> [w304]
          frame #0 {
            n200 = call "获取阵列信息.vi"("MB session in"=w296) -> ("error out"=w302:errorcluster, "阵列信息"=→"阵列信息":cluster{"阵列电压V":dbl, "阵列电流A":dbl, "发电功率W":dbl}, "MB session out"=w299:refnum<class "MB_Master.lvclass">)  [unwired: 8 in]
            n201 = call "获取蓄电池信息.vi"("error in (no error)"=w302, "MB session in"=w299) -> ("error out"=w301:errorcluster, "蓄电池信息"=→"蓄电池信息":T2, "MB session out"=w298:refnum<class "MB_Master.lvclass">)  [unwired: 7 in]
            n202 = call "获取直流负载信息.vi"("error in (no error)"=w301, "MB session in"=w298) -> ("error out"=w300:errorcluster, "直流负载信息"=→"直流负载信息":cluster{"负载电压V":dbl, "负载电流A":dbl, "负载功率W":dbl}, "MB session out"=w297:refnum<class "MB_Master.lvclass">)  [unwired: 7 in]
            n203 = call "获取控制器信息.vi"("error in (no error)"=w300, "MB session in"=w297) -> ("error out"=w291:errorcluster, "控制器信息"=→"控制器信息":cluster{"设备温度℃":dbl}, "MB session out"=w290:refnum<class "MB_Master.lvclass">)  [unwired: 7 in]
            n204 = call "获取充放电量信息.vi"("error in (no error)"=w291, "MB session in"=w290) -> ("error out"=w287:errorcluster, "充放电信息"=→"充放电信息":T1, "MB session out"=w288:refnum<class "MB_Master.lvclass">)  [unwired: 7 in]
            n205 = call "获取MPPT状态.vi"("error in (no error)"=w287, "MB session in"=w288) -> ("error out"=w286:errorcluster, "结果字符串"=→"状态":string)  [unwired: 6 in, 2 out]
          }
          frame #1 {
            n206 = Unbundle By Name(w304) -> ("status"=w305:bool)
            n207 = Not(x=w305) -> (.not. x?=w303:bool)
            "通讯状态 2" <- w303
            n208 = global write "通讯全局变量.vi" "MPPT-12 通讯状态"(w303) -> ()
          }
        }
      }
      frame "open" {
        n209 = local write "通讯状态 2"(FALSE ("通讯状态")) -> ()
        n210 = global read "通讯全局变量断电保存.vi" "MPPT-12 Serial"() -> (w311:refnum<visa-resource-name>)
        n211 = call "open Serial MB.vi"("Slave ID"=u8 1, "VISA Resource"=w311, "MB session in"=w309) -> ("error out"=w308:errorcluster, "MB session out"=w312:refnum<class "MB_Master.lvclass">)  [unwired: 7 in]
        n212 = global write "通讯全局变量.vi" "MPPT-12 MB session"(w312) -> ()
        n213 = case shown="错误" w308 {
          tunnel: [T12."Disabled and Grayed Out" ("禁用") T12."Enabled" ("禁用")] -> w307
          tunnel: [TRUE _] -> w306
          frame No Error {
          }
          frame Error {
          }
        }
        n214 = property on="MPPT-12 串口" class="VISAName"("DisabledEnum"=w307) -> ()  [unwired: 2 in, 2 out]
        n215 = property on="MPPT-12 启用" class="Bool (严格)"("Value"=w306) -> ()  [unwired: 2 in, 2 out]
      }
      frame "close" {
        n216 = local write "通讯状态 2"(FALSE ("通讯状态")) -> ()
        n217 = call "close MB.vi"("MB session in"=w319) -> ("error out"=w318:errorcluster)  [unwired: 10 in]
        n218 = case shown="无错误" w318 {
          frame No Error {
            n219 = property on="MPPT-12 串口" class="VISAName"("DisabledEnum"=T12."Enabled" ("禁用")) -> ()  [unwired: 2 in, 2 out]
          }
          frame Error {
          }
        }
      }
    }
  }
  n220 = while {
    tunnel: w7 -> [w332]
    tunnel: [w324] -> _
    shift-right: [w325] -> _
    shift-left: -1 ("超时毫秒(-1)") -> [w326]
    stop <- FALSE stop-if-true
    n221 = Dequeue Element(queue=w332, timeout in ms (-1)=w326) -> (element=w329:string, timed out?=w331:bool)  [unwired: 1 in, 2 out]
    n222 = Select(t="poll" ("元素"), s=w331, f=w329) -> (s? t:f=w328:string)
    n223 = global read "通讯全局变量.vi" "MPPT-24 MB session"() -> (w323:refnum<class "MB_Master.lvclass">)
    n224 = case shown="\"open\"" w328 {
      tunnel: [_ w337 w361 w371] -> w324
      tunnel: w326 -> [w333 w335 _ _]
      tunnel: [w333 w335 1000 ("超时毫秒(-1)") -1 ("超时毫秒(-1)")] -> w325
      tunnel: w323 -> [_ w334 w363 w373]
      frame Default {
      }
      frame "poll" {
        n225 = flat-sequence {
          tunnel: [w342] -> w336
          tunnel: w334 -> [w349]
          tunnel: [w357] -> w337
          tunnel: w336 -> [w357]
          frame #0 {
            n226 = call "获取阵列信息.vi"("MB session in"=w349) -> ("error out"=w355:errorcluster, "阵列信息"=→"阵列信息 2":cluster{"阵列电压V":dbl, "阵列电流A":dbl, "发电功率W":dbl}, "MB session out"=w352:refnum<class "MB_Master.lvclass">)  [unwired: 8 in]
            n227 = call "获取蓄电池信息.vi"("error in (no error)"=w355, "MB session in"=w352) -> ("error out"=w354:errorcluster, "蓄电池信息"=→"蓄电池信息 2":T2, "MB session out"=w351:refnum<class "MB_Master.lvclass">)  [unwired: 7 in]
            n228 = call "获取直流负载信息.vi"("error in (no error)"=w354, "MB session in"=w351) -> ("error out"=w353:errorcluster, "直流负载信息"=→"直流负载信息 2":cluster{"负载电压V":dbl, "负载电流A":dbl, "负载功率W":dbl}, "MB session out"=w350:refnum<class "MB_Master.lvclass">)  [unwired: 7 in]
            n229 = call "获取控制器信息.vi"("error in (no error)"=w353, "MB session in"=w350) -> ("error out"=w343:errorcluster, "控制器信息"=→"控制器信息 2":cluster{"设备温度℃":dbl}, "MB session out"=w341:refnum<class "MB_Master.lvclass">)  [unwired: 7 in]
            n230 = call "获取充放电量信息.vi"("error in (no error)"=w343, "MB session in"=w341) -> ("error out"=w344:errorcluster, "充放电信息"=→"充放电信息 2":T1, "MB session out"=w340:refnum<class "MB_Master.lvclass">)  [unwired: 7 in]
            n231 = call "获取MPPT状态.vi"("error in (no error)"=w344, "MB session in"=w340) -> ("error out"=w342:errorcluster, "结果字符串"=→"状态 2":string)  [unwired: 6 in, 2 out]
          }
          frame #1 {
            n232 = Unbundle By Name(w357) -> ("status"=w358:bool)
            n233 = Not(x=w358) -> (.not. x?=w356:bool)
            "通讯状态 3" <- w356
            n234 = global write "通讯全局变量.vi" "MPPT-24 通讯状态"(w356) -> ()
          }
        }
      }
      frame "open" {
        n235 = local write "通讯状态 3"(FALSE ("通讯状态")) -> ()
        n236 = global read "通讯全局变量断电保存.vi" "MPPT-24 Serial"() -> (w365:refnum<visa-resource-name>)
        n237 = call "open Serial MB.vi"("Slave ID"=u8 2, "VISA Resource"=w365, "MB session in"=w363) -> ("error out"=w361:errorcluster, "MB session out"=w366:refnum<class "MB_Master.lvclass">)  [unwired: 7 in]
        n238 = global write "通讯全局变量.vi" "MPPT-24 MB session"(w366) -> ()
        n239 = case shown="无错误" w361 {
          tunnel: [T12."Disabled and Grayed Out" ("禁用") T12."Enabled" ("禁用")] -> w360
          tunnel: [TRUE ("MPPT-24 启用") _] -> w359
          frame No Error {
          }
          frame Error {
          }
        }
        n240 = property on="MPPT-24 串口" class="VISAName"("DisabledEnum"=w360) -> ()  [unwired: 2 in, 2 out]
        n241 = property on="MPPT-24 启用" class="Bool (严格)"("Value"=w359) -> ()  [unwired: 2 in, 2 out]
      }
      frame "close" {
        n242 = local write "通讯状态 3"(FALSE ("通讯状态")) -> ()
        n243 = call "close MB.vi"("MB session in"=w373) -> ("error out"=w371:errorcluster)  [unwired: 10 in]
        n244 = case shown="无错误" w371 {
          frame No Error {
            n245 = property on="MPPT-24 串口" class="VISAName"("DisabledEnum"=T12."Enabled" ("禁用")) -> ()  [unwired: 2 in, 2 out]
          }
          frame Error {
          }
        }
      }
    }
  }
  n246 = while {
    tunnel: w11 -> [w384]
    tunnel: [w376] -> _
    shift-right: [w377] -> _
    shift-left: -1 ("超时毫秒(-1)") -> [w378]
    stop <- FALSE stop-if-true
    n247 = Dequeue Element(queue=w384, timeout in ms (-1)=w378) -> (element=w381:string, timed out?=w383:bool)  [unwired: 1 in, 2 out]
    n248 = Select(t="poll" ("元素"), s=w383, f=w381) -> (s? t:f=w380:string)
    n249 = case shown="\"close\"" w380 {
      tunnel: [_ w388 w411 w413] -> w376
      tunnel: w378 -> [w385 w386 _ _]
      tunnel: [w385 w386 1000 ("超时毫秒(-1)") -1 ("超时毫秒(-1)")] -> w377
      frame Default {
      }
      frame "poll" {
        n250 = flat-sequence {
          tunnel: [w397] -> w387
          tunnel: [w406] -> w388
          tunnel: w387 -> [w406]
          frame #0 {
            n251 = global read "通讯全局变量.vi" "ZLAN 6842 MB session"() -> (w396:refnum<class "MB_Master.lvclass">)
            n252 = call "获取DI状态.vi"("MB session in"=w396) -> ("error out"=w394:errorcluster, "Coils"=w390:bool[], "MB session out"=w395:refnum<class "MB_Master.lvclass">)  [unwired: 8 in]
            n253 = call "获取DO状态.vi"("error in (no error)"=w394, "MB session in"=w395) -> ("error out"=w393:errorcluster, "Coils"=w391:bool[], "MB session out"=w392:refnum<class "MB_Master.lvclass">)  [unwired: 7 in]
            n254 = call "获取AI状态.vi"("error in (no error)"=w393, "MB session in"=w392) -> ("error out"=w397:errorcluster, "Registers"=w399:u16[])  [unwired: 7 in, 1 out]
            n255 = case shown="无错误" w397 {
              tunnel: w399 -> [w402 _]
              tunnel: w391 -> [w401 _]
              tunnel: w390 -> [w400 _]
              frame No Error {
                n256 = global write "通讯全局变量.vi" "DO"(w401) -> ()
                n257 = global write "通讯全局变量.vi" "DI"(w400) -> ()
                n258 = global read "通讯全局变量断电保存.vi" "工程量转换"() -> (w404:T11)
                n259 = Array To Cluster(array=w402) -> (cluster=w405:T13)
                n260 = call "原始值工程转换.vi"("工程量转换"=w404, "AD当前原始值"=w405) -> ("AD当前转换值"=w403:T5)  [unwired: 9 in]
                n261 = global write "通讯全局变量.vi" "AD当前原始值"(w405) -> ()
                n262 = global write "通讯全局变量.vi" "AD当前转换值"(w403) -> ()
              }
              frame Error {
              }
            }
            n263 = Unbundle By Name(w397) -> ("status"=w398:bool)
            n264 = Not(x=w398) -> (.not. x?=w389:bool)
            "通讯状态" <- w389
            n265 = global write "通讯全局变量.vi" "ZLAN 通讯状态"(w389) -> ()
          }
          frame #1 {
          }
        }
      }
      frame "open" {
        n266 = local write "通讯状态"(FALSE ("通讯状态")) -> ()
        n267 = global read "通讯全局变量.vi" "ZLAN 6842 MB session"() -> (w409:refnum<class "MB_Master.lvclass">)
        n268 = global read "通讯全局变量断电保存.vi" "ZLAN IP"() -> (w407:string)
        n269 = call "open TCP MB.vi"("IP Address"=w407, "MB session in"=w409) -> ("error out"=w411:errorcluster, "MB session out"=w408:refnum<class "MB_Master.lvclass">)  [unwired: 8 in]
        n270 = global write "通讯全局变量.vi" "ZLAN 6842 MB session"(w408) -> ()
      }
      frame "close" {
        n271 = local write "通讯状态"(FALSE ("通讯状态")) -> ()
        n272 = global read "通讯全局变量.vi" "ZLAN 6842 MB session"() -> (w415:refnum<class "MB_Master.lvclass">)
        n273 = call "close MB.vi"("MB session in"=w415) -> ("error out"=w414:errorcluster)  [unwired: 10 in]
        n274 = call "时间延迟3"("error in (no error)"=w414) -> ("error out"=w413:errorcluster)  [unwired: 10 in]
      }
    }
  }
  n275 = while {
    stop <- FALSE stop-if-true
    # "环境变量信息传输"
    n276 = global read "通讯全局变量.vi" "环境变量"() -> (w422:T4)
    n277 = Wait (ms)(milliseconds to wait=u32 1000 ("等待时间（毫秒）")) -> ()  [unwired: 1 out]
    n278 = Unbundle By Name(w422) -> ("蓄电池电压"=w421:dbl, "室温"=w420:dbl, "湿度"=w419:dbl)
    n279 = global read "气象全局变量.vi" "环境变量"() -> (w423:cluster{"电压":dbl, "室温":dbl, "湿度":dbl})
    n280 = Bundle By Name(cluster=w423, "电压"=w421, "室温"=w420, "湿度"=w419) -> (w424:cluster{"电压":dbl, "室温":dbl, "湿度":dbl})
    n281 = global write "气象全局变量.vi" "环境变量"(w424) -> ()
  }
